vi "LVClass_ClosedLoopSmoothing_SetData.vi"(0 "ClosedLoopSmoothing in":refnum<class "ClosedLoopSmoothing.lvclass">, 5 "CLoopSmoothingParams":T1, 11 "error in (no error)":errorcluster) -> (4 "ClosedLoopSmoothing out":refnum<class "ClosedLoopSmoothing.lvclass">, 15 "error out":errorcluster)   [LabVIEW 2020, in "ClosedLoopSmoothing.lvclass"]
doc: "Set closed loop smoothing parameters.\n\n<B>smoothing_paramsIn</B> : Closed Loop smoothing params object.\n<B>smoothing_paramsOut</B> : Closed Loop smoothing params object.\n<B>low_gain_factor</B> : lowest value for gain factor\n<B>high_gain_factor</B> : highest value for gain factor\n<B>low_amplitude</B> : lowest amplitude value before switching to linear behavior\n<B>high_amplitude</B> : highest amplitude value where linear behavior stops"
uses:
  ClosedLoopSmoothing.lvclass
  ClosedLoopSmoothingParameters.ctl
  ClosedLoopSmoothing.lvclass/ClosedLoopSmoothing.ctl
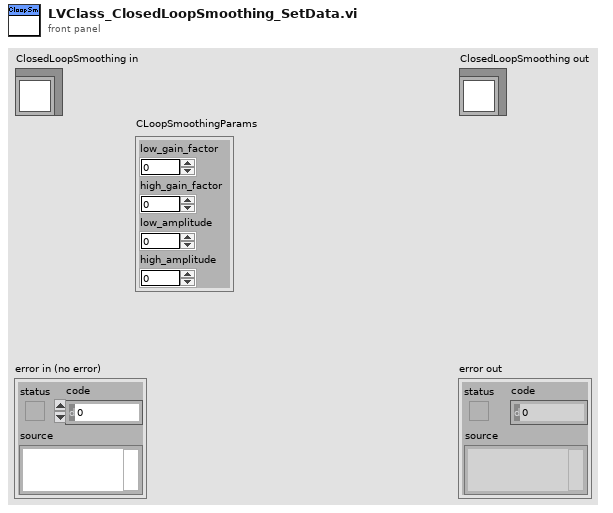
[diagram p1: front panel]
types:
  T1 = typedef "ClosedLoopSmoothingParameters.ctl" = cluster{"low_gain_factor":sgl, "high_gain_factor":sgl, "low_amplitude":i32, "high_amplitude":i32}
  T2 = typedef "ClassID.ctl" = i64
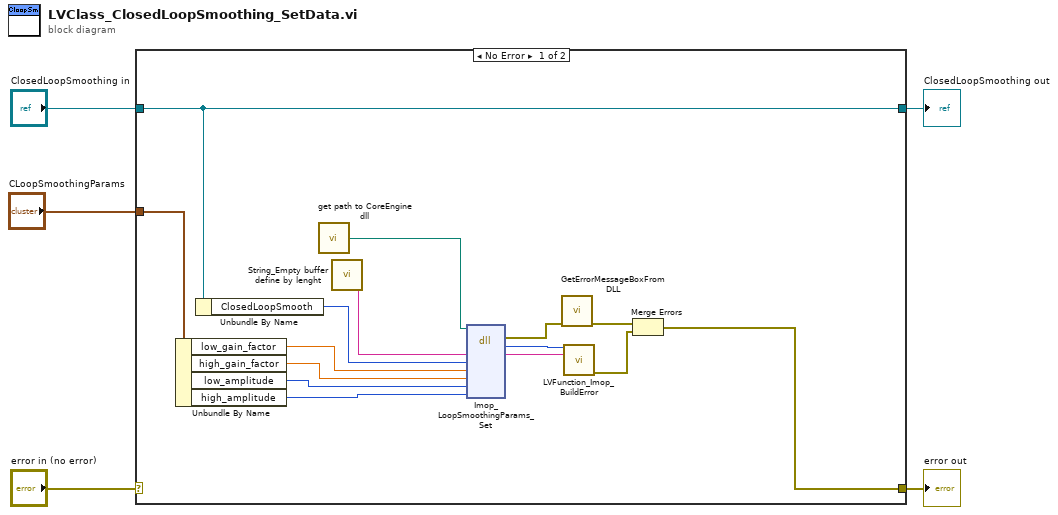
[diagram p0: block diagram]
diagram:
  n1 = case shown="No Error" "error in (no error)" {
    selector: "error in (no error)" -> [_ w22]
    tunnel: [w13 w22] -> w4
    tunnel: [w6 w21] -> w2
    tunnel: "ClosedLoopSmoothing in" -> [w6 w21]
    tunnel: "CLoopSmoothingParams" -> [w12 _]
    frame No Error {
      n2 = Unbundle By Name(w12) -> ("low_gain_factor"=w11:sgl, "high_gain_factor"=w10:sgl, "low_amplitude"=w9:i32, "high_amplitude"=w8:i32)
      n3 = Unbundle By Name(w6) -> ("ClosedLoopSmooth"=w7:T2)
      n4 = call "get path to CoreEngine dll.vi"() -> ("path to wavekit library"=w14:path)  [unwired: 14 in, 1 out]
      n5 = call "String_Empty buffer define by lenght.vi"() -> ("Empty buffer"=w20:string)  [unwired: 1 in]
      n6 = dll-call lib="D:/soft/HASO_v3/SVN_trunk/ImOpCoreEngine4_LV2011/DLLs/c_interface_vc100.dll" fn="Imop_LoopSmoothingParams_Set"(path in=w14, "message"=w20, "smoothing_params"=w7, "low_gain_factor"=w11, "high_gain_factor"=w10, "low_amplitude"=w9, "High_amplitude"=w8) -> (error out=w17:errorcluster, "return type"=w18:i32, "message"=w19:string)  [unwired: 7 in, 1 out]
      n7 = call "GetErrorMessageBoxFromDLL.vi"("error IN"=w17) -> ("error OUT"=w16:errorcluster)  [unwired: 10 in]
      n8 = call "LVFunction_Imop_BuildError.vi"("code"=w18, "String to Prepend to source (\"\")"=w19) -> ("error out"=w15:errorcluster)  [unwired: 13 in]
      n9 = Merge Errors(w16, w15) -> (w13:errorcluster)
    }
    frame Error {
    }
  }
  "error out" <- w4
  "ClosedLoopSmoothing out" <- w2
